vi "decimalToBinary.vi"(1 "decimal input":u8 max=3 step=1) -> (0 "Binary out":cluster{"CTRL2":u8, "CTRL1":u8})   [LabVIEW 2020]
panel:
  out "reversed decimal":u8
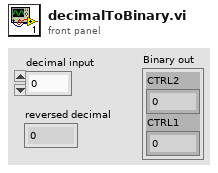
[diagram p1: front panel]
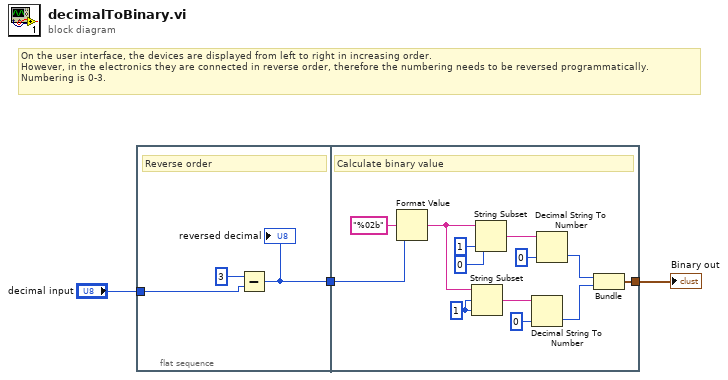
[diagram p0: block diagram]
diagram:
  # "On the user interface, the devices are displayed from left to right in increasing order. \nHowever, in the electronics they are connected in reverse order, therefore the numbering needs to be reversed programmatically.\nNumbering is 0-3."
  n1 = flat-sequence {
    tunnel: "decimal input" -> [w4]
    tunnel: [w6] -> w1
    tunnel: [w7] -> w2
    tunnel: w1 -> [w18]
    frame #0 {
      # "Reverse order"
      n2 = Subtract(x=u8 3, y=w4) -> (x-y=w6:u8)
      "reversed decimal" <- w6
    }
    frame #1 {
      w15 = 1 ("length (rest)")
      # "Calculate binary value"
      n3 = Format Value(format string="%02b", value (0)=w18) -> (output string=w16:string)  [unwired: 1 in]
      n4 = String Subset(string=w16, offset (0)=w15, length (rest)=w15) -> (substring=w10:string)
      n5 = String Subset(string=w16, offset (0)=0, length (rest)=1 ("length (rest)")) -> (substring=w13:string)
      n6 = Decimal String To Number(string=w10, default (0L)=u8 0 ("default (0 I32)")) -> (number=w8:u8)  [unwired: 1 in, 1 out]
      n7 = Decimal String To Number(string=w13, default (0L)=u8 0 ("default (0 I32)")) -> (number=w9:u8)  [unwired: 1 in, 1 out]
      n8 = Bundle(w9, w8) -> (w7:cluster{u8, u8})  [unwired: 1 in]
    }
  }
  "Binary out" <- w2
